vi "ACR_APX_Initialize.vi"(9 "Numeric":i32, 10 "Array":string[][](array[string]), 11 "Automation Refnum in":refnum<k7>) -> ()   [LabVIEW 2015]
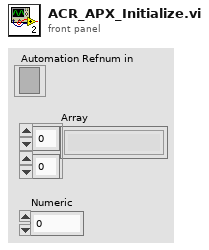
[diagram p1: front panel]
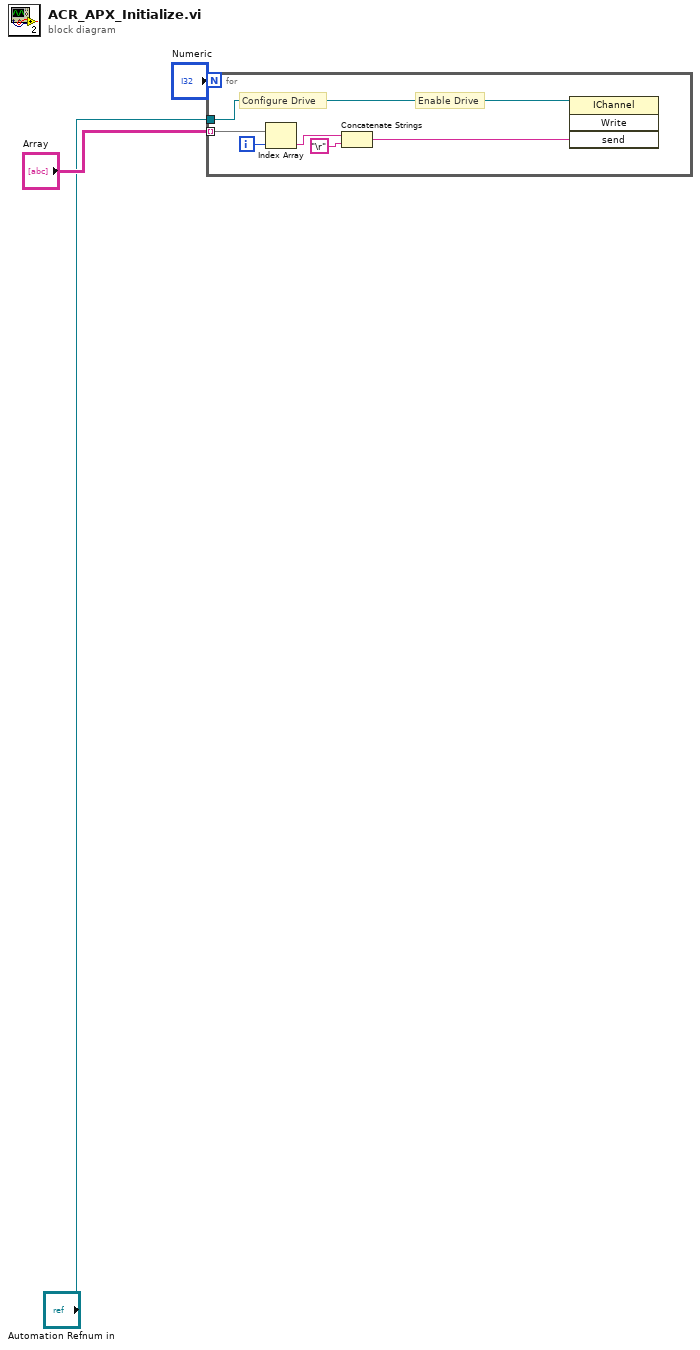
[diagram p0: block diagram]
diagram:
  n1 = for {
    N: "Numeric" -> [_]
    tunnel: "Automation Refnum in" -> [w5]
    tunnel: "Array" -> [w4] mode=indexing
    i -> [w6]
    # "Enable Drive"
    # "Configure Drive"
    n2 = Index Array(array=w4, index=w6) -> (element=w8:string)
    n3 = Concatenate Strings(w8, "\r") -> (w9:string)
    n4 = invoke class="IChannel" method="Write"(reference=w5, "send"=w9) -> ()  [unwired: 2 in, 4 out]
  }
